vi "LEIN Full cluster pack out if ACTI 6.vi"(7 "element":T3={"CMD"={"SID"=0, "ANF"=FALSE, "CMD"=enum."TASK", "DATA"=[]}, "Retry if  unsucessful"=FALSE, "LEIN reply holder"={"Reply msg(cmdif no reply)"={"SID"=0, "ANF"=FALSE, "CMD"=enum."TASK", "DATA"=[]}, "Reply time"=timestamp(0 s since 1904-01-01), "Valid reply"=FALSE}, "Reply in custom Q"=FALSE, "LEIN custom reply Q"=refnum}, 11 "error in (no error)":errorcluster) -> (3 "Valid replay":bool, 4 "ANF":bool, 6 "SID":u8, 8 "Reply":T1, 10 "CMD":T1={"SID"=0, "ANF"=FALSE, "CMD"=enum."TASK", "DATA"=[]}, 15 "error out":errorcluster)   [LabVIEW 2011]
uses:
  Defenitions/LEIN CMD Cluster.ctl
  Defenitions/LEIN CMD List.ctl
  Defenitions/LEIN cycle holder.ctl
  Defenitions/LEIN Reply Holder.ctl
  Defenitions/LEIN custom reply Q.ctl
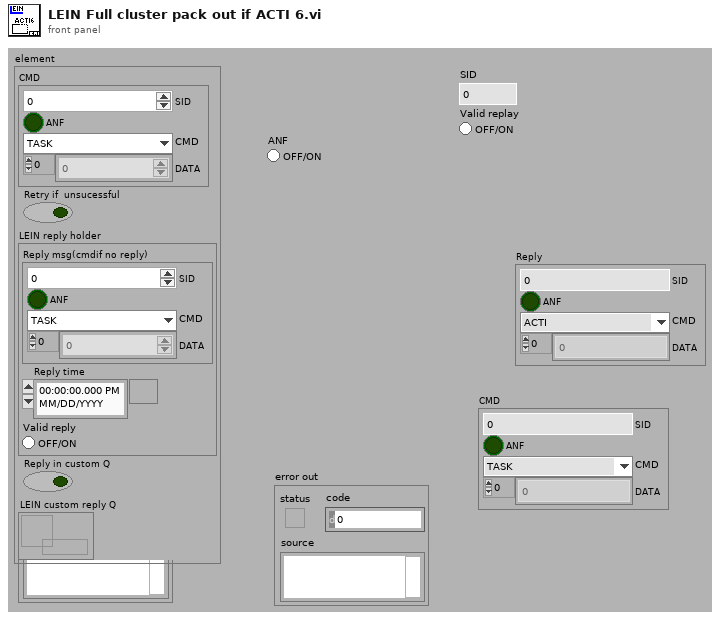
[diagram p1: front panel]
types:
  T1 = typedef "LEIN CMD Cluster.ctl" = cluster{"SID":u8, "ANF":bool, "CMD":T2, "DATA":u8[]}
  T2 = typedef "LEIN CMD List.ctl" = enum8{"ACTI", "TASK", "RES0", "STAT", "RES1", "RES2", "RES3", "USER"}
  T3 = typedef "LEIN cycle holder.ctl" = cluster{"CMD":T1, "Retry if  unsucessful":bool, "LEIN reply holder":T4, "Reply in custom Q":bool, "LEIN custom reply Q":T5}
  T4 = typedef "LEIN Reply Holder.ctl" = cluster{"Reply msg(cmdif no reply)":T1, "Reply time":timestamp, "Valid reply":bool}
  T5 = typedef "LEIN custom reply Q.ctl" = refnum<queue>
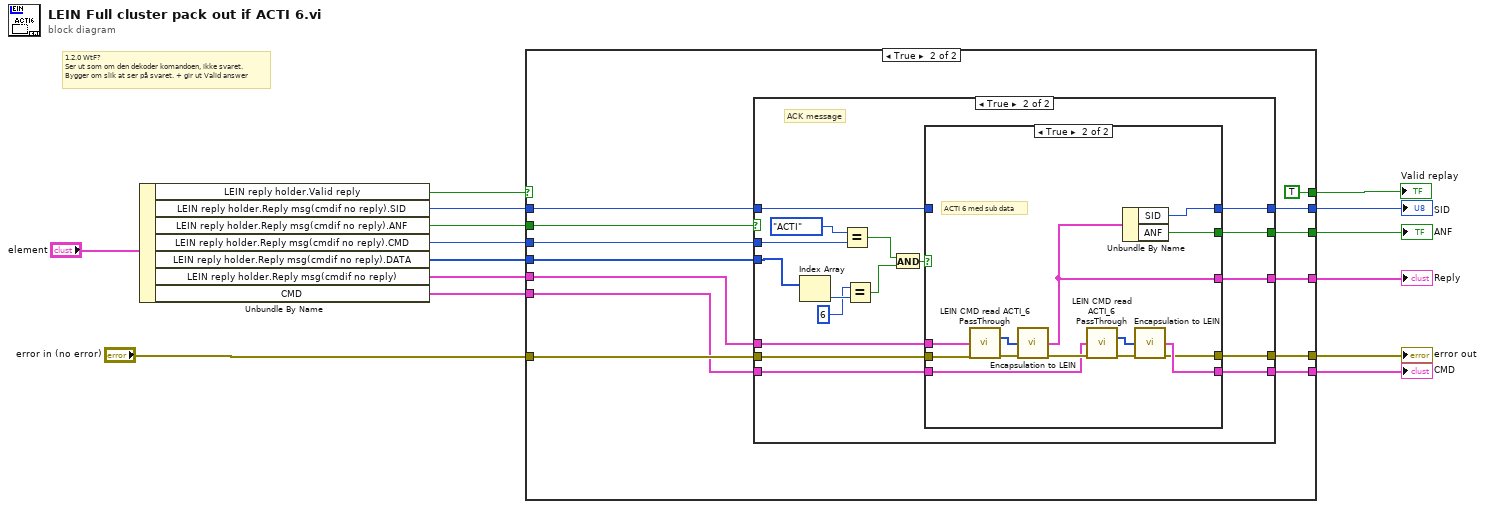
[diagram p0: block diagram]
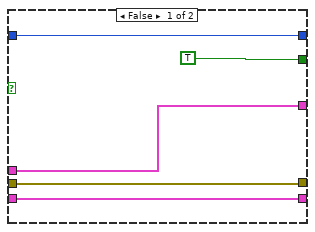
[diagram p4: hidden frame]
diagram:
  # "1.2.0 WtF? \nSer ut som om den dekoder komandoen, ikke svaret.\nBygger om slik at ser på svaret. + gir ut Valid answer"
  n1 = Unbundle By Name("element") -> ("LEIN reply holder.Valid reply"=w2:bool, "LEIN reply holder.Reply msg(cmdif no reply).SID"=w6:u8, "LEIN reply holder.Reply msg(cmdif no reply).ANF"=w11:bool, "LEIN reply holder.Reply msg(cmdif no reply).CMD"=w7:T2, "LEIN reply holder.Reply msg(cmdif no reply).DATA"=w8:u8[], "LEIN reply holder.Reply msg(cmdif no reply)"=w10:T1, "CMD"=w4:T1)
  n2 = case shown="True" w2 {
    selector: w2 -> [w16 _]
    tunnel: [_ w33] -> w15
    tunnel: [w18 w32] -> w14
    tunnel: [w20 w31] -> w13
    tunnel: "error in (no error)" -> [w20 w30]
    tunnel: w11 -> [_ w29]
    tunnel: w10 -> [w18 w28]
    tunnel: w8 -> [_ w27]
    tunnel: w7 -> [_ w26]
    tunnel: w6 -> [w17 w25]
    tunnel: [w17 w24] -> w5
    tunnel: w4 -> [w19 w23]
    tunnel: [w19 w22] -> w3
    tunnel: [w16 TRUE] -> w1
    frame False {
    }
    frame True {
      n3 = case shown="True" w29 {
        selector: w29 -> [w38 _]
        tunnel: w26 -> [_ w52]
        tunnel: w27 -> [_ w55]
        tunnel: w28 -> [w35 w47]
        tunnel: w30 -> [w37 w46]
        tunnel: [w37 w45] -> w31
        tunnel: [w35 w44] -> w32
        tunnel: [w38 w43] -> w33
        tunnel: w25 -> [w36 w42]
        tunnel: [w36 w41] -> w24
        tunnel: w23 -> [w34 w40]
        tunnel: [w34 w39] -> w22
        frame False {
        }
        frame True {
          # "ACK message"
          n4 = Index Array(array=w55) -> (element=w54:u8)  [unwired: 1 in]
          n5 = Equal?(x=LEIN_CMD_List."ACTI", y=w52) -> (x = y?=w50:bool)
          n6 = Equal?(x=u8 6, y=w54) -> (x = y?=w49:bool)
          n7 = And(x=w50, y=w49) -> (x .and. y?=w48:bool)
          n8 = case shown="True" w48 {
            tunnel: w47 -> [w59 w73]
            tunnel: w46 -> [w60 w70]
            tunnel: [w60 w61] -> w45
            tunnel: [w59 w67] -> w44
            tunnel: [TRUE ("ANF") w69] -> w43
            tunnel: w42 -> [w57 _]
            tunnel: [w57 w68] -> w41
            tunnel: w40 -> [w56 w63]
            tunnel: [w56 w62] -> w39
            frame False {
            }
            frame True {
              # "ACTI 6 med sub data"
              n9 = call "LEIN CMD read ACTI_6 PassThrough.vi"("CMD"=w73, "error in (no error)"=w70) -> ("Reply from sub ID"=w72:u8[], "error out"=w71:errorcluster)  [unwired: 10 in, 2 out]
              n10 = call "Encapsulation to LEIN.vi"("Data and header"=w72, "error in (no error)"=w71) -> ("CMD out"=w67:T1, "error out"=w64:errorcluster)  [unwired: 10 in, 2 out]
              n11 = call "LEIN CMD read ACTI_6 PassThrough.vi"("CMD"=w63, "error in (no error)"=w64) -> ("Reply from sub ID"=w65:u8[], "error out"=w66:errorcluster)  [unwired: 10 in, 2 out]
              n12 = Unbundle By Name(w67) -> ("SID"=w68:u8, "ANF"=w69:bool)
              n13 = call "Encapsulation to LEIN.vi"("Data and header"=w65, "error in (no error)"=w66) -> ("CMD out"=w62:T1, "error out"=w61:errorcluster)  [unwired: 10 in, 2 out]
            }
          }
        }
      }
    }
  }
  "ANF" <- w15
  "Reply" <- w14
  "error out" <- w13
  "SID" <- w5
  "CMD" <- w3
  "Valid replay" <- w1
